vi "Shutdown.vi"(8 "error in (no error)":errorcluster, 11 "Actor API in":refnum<class "Actor API.lvclass">) -> (0 "error out":errorcluster)   [LabVIEW 2020, in "Actor API.lvclass"]
uses:
  Actor API.lvclass
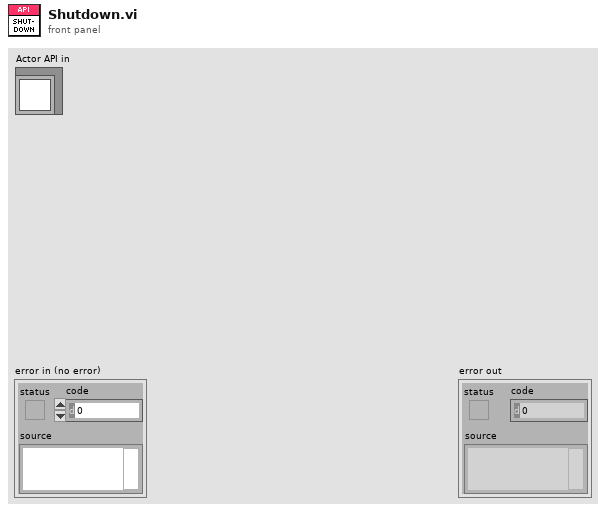
[diagram p1: front panel]
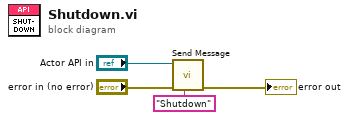
[diagram p0: block diagram]
diagram:
  n1 = call "Send Message.vi"("Name"="Shutdown", "error in (no error)"="error in (no error)", "Actor API in"="Actor API in") -> ("error out"=→"error out":errorcluster)  [unwired: 8 in]
